vi "StringArray to ByteArray.vi"(1 "String Len":u8, 2 "String":string[](array[string])) -> (0 "Byte Array":u8[](array[numeric]))   [LabVIEW 2014, in "Simatic S7.lvlib"]
uses:
  Simatic S7.lvlib
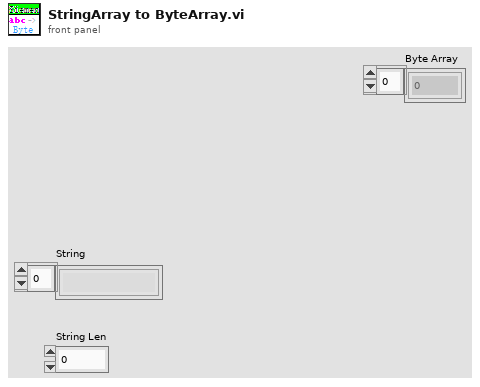
[diagram p1: front panel]
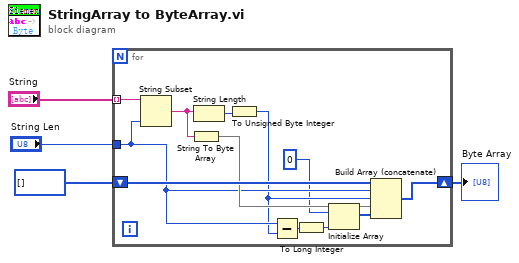
[diagram p0: block diagram]
diagram:
  n1 = for {
    tunnel: "String" -> [w16] mode=indexing
    tunnel: "String Len" -> [w10]
    shift-right: [w12] -> w1
    shift-left: u8[] [] -> [w13]
    n2 = String Subset(string=w16, length (rest)=w10) -> (substring=w14:string)  [unwired: 1 in]
    n3 = String To Byte Array(string=w14) -> (unsigned byte array=w11:u8[])
    n4 = String Length(string=w14) -> (length=w15:i32)
    n5 = To Unsigned Byte Integer(number=w15) -> (unsigned 8bit integer=w9:u8)
    n6 = Subtract(x=w10, y=w9) -> (x-y=w6:u8)
    n7 = To Long Integer(number=w6) -> (32bit integer=w5:i32)
    n8 = Initialize Array(u8 0, w5) -> (w8:u8[])
    n9 = Build Array (concatenate)(w13, w10, w9, w11, w8) -> (w12:u8[])
  }
  "Byte Array" <- w1
